vi "calculator_ES_main.vi"() -> ()   [LabVIEW 2020]
uses:
  #typedef_ProgramData.ctl
  #typedef_Tab_buttons.ctl
panel:
  in  "Program Data":T1
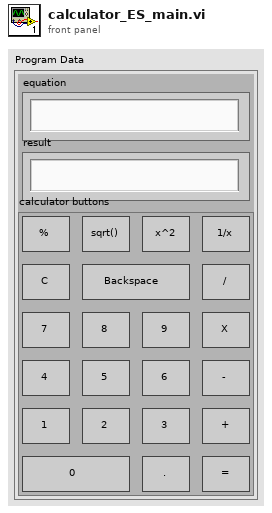
[diagram p1: front panel]
types:
  T1 = typedef "#typedef_ProgramData.ctl" = cluster{"equation":string, "result":string, "calculator buttons":T2}
  T2 = typedef "#typedef_Tab_buttons.ctl" = cluster{bool, bool, bool, bool, bool, bool, bool, bool, bool, bool, bool, bool, bool, bool, bool, bool, bool, bool, bool, bool, bool, bool}
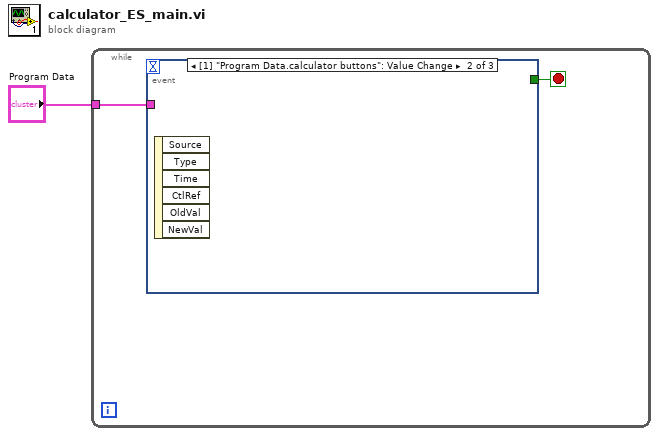
[diagram p0: block diagram]
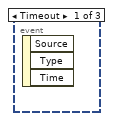
[diagram p2: hidden frame]
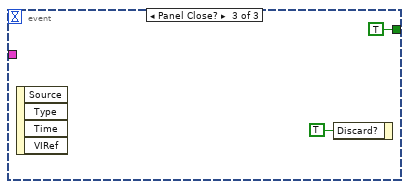
[diagram p3: hidden frame]
diagram:
  n1 = while {
    tunnel: "Program Data" -> [w3]
    stop <- w2 stop-if-true
    n2 = event shown="[1] \"Program Data.calculator buttons\": Value Change" {
      selector: _ -> [_ _ _]
      dyn-events: _ -> [_ _ _]
      timeout: _ -> [_ _ _]
      tunnel: w3 -> [_ _ _]
      tunnel: [_ _ TRUE] -> w2
      event Timeout {
        n3 = event-data() -> ()  [unwired: 1 in, 3 out]
      }
      event Value Change {
        n4 = event-data() -> ()  [unwired: 1 in, 6 out]
      }
      event Panel Close? {
        n5 = event-data() -> ()  [unwired: 1 in, 4 out]
        n6 = event-data("Discard?"=TRUE) -> ()  [unwired: 1 in, 1 out]
      }
    }
  }
